vi "Disconnect Connection.vi"(8 "error in (no error)":errorcluster, 11 "NodeRed-LV-Interface in":refnum<class "NodeRed-LV-Interface.lvclass">) -> (0 "error out":errorcluster, 3 "NodeRed-LV-Interface out":refnum<class "NodeRed-LV-Interface.lvclass">)   [LabVIEW 2020, in "NodeRed-LV-Interface.lvclass"]
uses:
  NodeRed-LV-Interface.lvclass
  NodeRed-LV-Interface.lvclass/NodeRed-LV-Interface.ctl
  <vilib>/event_ctls.llb/usereventprio.ctl
  ab26f5f1-ecbb-4796-8587-aac71bc4746e.vi
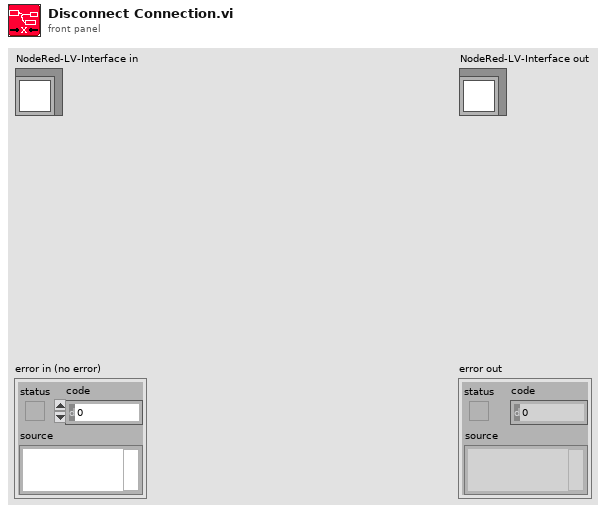
[diagram p1: front panel]
types:
  T1 = typedef "usereventprio.ctl" = enum32{"high priority", "normal priority"}
  T2 = cluster{"Send data":refnum<user-event>, "Receive data":refnum<user-event>, "IP Address":string, "Port":u16, "Stop Event":refnum<user-event>, "UDP Engine":refnum<vi>}
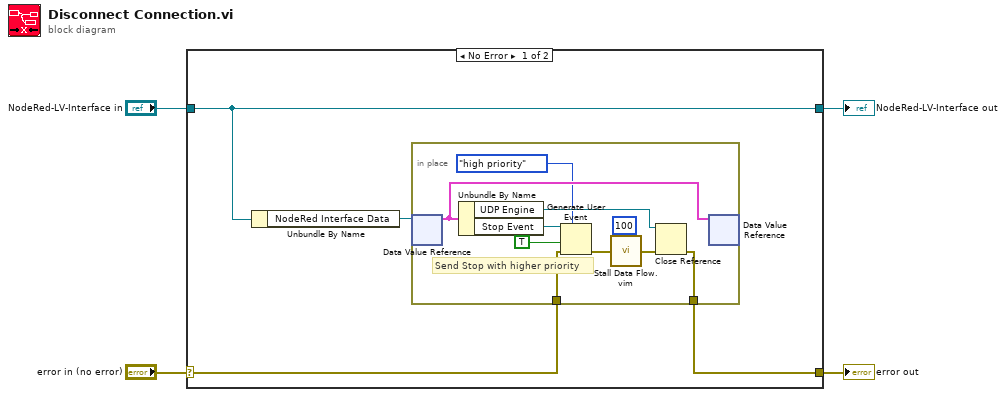
[diagram p0: block diagram]
diagram:
  n1 = case shown="No Error" "error in (no error)" {
    selector: "error in (no error)" -> [w6 w20]
    tunnel: [w5 w20] -> w3
    tunnel: [w8 w19] -> w1
    tunnel: "NodeRed-LV-Interface in" -> [w8 w19]
    frame No Error {
      n2 = Unbundle By Name(w8) -> ("NodeRed Interface Data"=w7:refnum<data-value>)
      n3 = in-place {
        in-place-border: w6 -> [w15]
        in-place-border: [w14] -> w5
        # "Send Stop with higher priority"
        n4 = in-place-dvr #1(w7) -> (w16:T2)  [unwired: 1 out]
        n5 = Unbundle By Name(w16) -> ("UDP Engine"=w17:refnum<vi>, "Stop Event"=w18:refnum<user-event>)
        n6 = Generate User Event(priority (normal)=usereventprio."high priority", user event=w18, event data cluster=TRUE ("event data"), error in=w15) -> (error out=w12:errorcluster)  [unwired: 1 out]
        n7 = call "Stall Data Flow.vim"("value in"=w12, "milliseconds to wait"=u32 100) -> ("value out"=w11:errorcluster)  [unwired: 1 out]
        n8 = Close Reference(reference=w17, error in (no error)=w11) -> (error out=w14:errorcluster)
        n9 = in-place-dvr #1(w16) -> ()  [unwired: 2 out]
      }
    }
    frame Error {
    }
  }
  "error out" <- w3
  "NodeRed-LV-Interface out" <- w1
